vi "DB_WriteInGen.vi"(8 "error in (no error)":errorcluster, 9 "Equipo_Medicion":T2, 10 "ID_MEDICION":i32, 11 "DB in":T1) -> (0 "error out":errorcluster, 3 "closeDB":T1[](array[typedef]))   [LabVIEW 2018]
uses:
  <vilib>/addons/database/Connection.llb/Conn ObjectReference.ctl
  Controls/Equipos_Medicion_cluster.ctl
  <vilib>/addons/database/NI_Database_API.lvlib
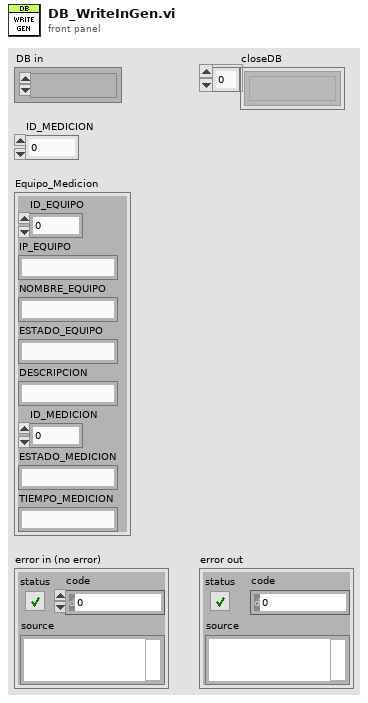
[diagram p1: front panel]
types:
  T1 = typedef "NI_Database_API.lvlib/Conn ObjectReference.ctl" = refnum<k1>
  T2 = typedef "Equipos_Medicion_cluster.ctl" = cluster{"ID_EQUIPO":i32, "IP_EQUIPO":string, "NOMBRE_EQUIPO":string, "ESTADO_EQUIPO":string, "DESCRIPCION":string, "ID_MEDICION":i32, "ESTADO_MEDICION":string, "TIEMPO_MEDICION":string}
  T3 = typedef "Cluster_Data.ctl" = cluster{"Equipo_Medicion":T2, "VIF_cluster":T4, "Power_cluster":T5, "THD_cluster":T6, "Polar_cluster":T7}
  T4 = typedef "VIF_cluster.ctl" = cluster{"VL_VL":cluster{"V1_V2":sgl, "V2_V3":sgl, "V3_V1":sgl, "Avg_VL_VL":sgl}, "IL_IL":cluster{"I1":sgl, "I2":sgl, "I3":sgl, "Avg_Amps":sgl}, "Frecuency":sgl, "Avg_Frecuency":sgl}
  T5 = typedef "Power_cluster.ctl" = cluster{"Real Power (kW)":cluster{"L1_kW":sgl, "L2_kW":sgl, "L3_kW":sgl, "Total_kW":sgl}, "Reactive Power (kVAR)":cluster{"L1_kVAR":sgl, "L2_kVAR":sgl, "L3_kVAR":sgl, "Total_kVAR":sgl}, "Aparent Power (kVA)":cluster{"L1_kVA":sgl, "L2_kVA":sgl, "L3_kVA":sgl, "Total_kVA":sgl}, "Power Factor (%)":cluster{"L1_PF":sgl, "L2_PF":sgl, "L3_PF":sgl, "Total_PF":sgl}}
  T6 = typedef "THD_cluster.ctl" = cluster{"V_THD":cluster{"Avg_V_V_THD":sgl, "V3_V1_THD":sgl, "V2_V3_THD":sgl, "V1_V2_THD":sgl}, "I_THD":cluster{"Avg_I_THD":sgl, "I4_THD":sgl, "I3_THD":sgl, "I2_THD":sgl, "I1_THD":sgl}}
  T7 = typedef "Polar_cluster.ctl" = cluster{"V_polar":cluster{"V1_ang":sgl, "V1_mag":sgl, "V2_ang":sgl, "V2_mag":sgl, "V3_ang":sgl, "V3_mag":sgl}, "I_polar":cluster{"I1_ang":sgl, "I1_mag":sgl, "I2_ang":sgl, "I2_mag":sgl, "I3_ang":sgl, "I3_mag":sgl}}
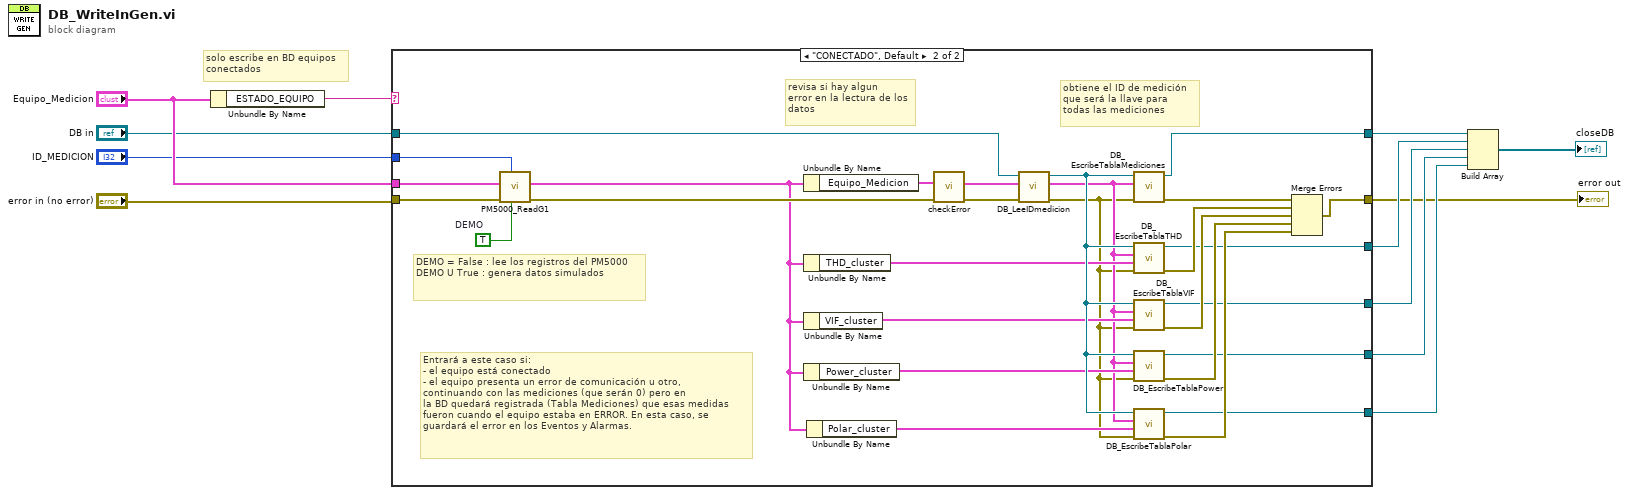
[diagram p0: block diagram]
diagram:
  # "solo escribe en BD equipos\nconectados"
  n1 = Unbundle By Name("Equipo_Medicion") -> ("ESTADO_EQUIPO"=w5:string)
  n2 = case shown="\"CONECTADO\", Default" w5 {
    tunnel: "error in (no error)" -> [w14 w42]
    tunnel: "DB in" -> [w13 w39]
    tunnel: "ID_MEDICION" -> [_ w41]
    tunnel: [w14 w38] -> w2
    tunnel: [w13 w19] -> w7
    tunnel: "Equipo_Medicion" -> [_ w40]
    tunnel: [_ w18] -> w11
    tunnel: [_ w17] -> w10
    tunnel: [_ w16] -> w9
    tunnel: [_ w15] -> w8
    frame "DESCONECTADO" {
      # "Equipo está deconectado"
    }
    frame "CONECTADO", Default {
      w36 = TRUE  # DEMO
      # "Entrará a este caso si:\n- el equipo está conectado\n- el equipo presenta un error de comunicación u otro,\ncontinuando con las mediciones (que serán 0) pero en\nla BD quedará registrada (Tabla Mediciones) que esas medidas\nfueron cuando el equipo estaba en ERROR. En esta caso, se \nguardará el error en los Eventos y Alarmas."
      # "obtiene el ID de medición\nque será la llave para \ntodas las mediciones"
      # "revisa si hay algun \nerror en la lectura de los\ndatos"
      # "DEMO = False : lee los registros del PM5000\nDEMO U True : genera datos simulados"
      n3 = call "PM5000_ReadG1.vi"("DEMO"=w36, "ID_MEDICION"=w41, "error in (no error)"=w42, "Equipo_Medicion"=w40) -> ("error out"=w37:errorcluster, "PM_out"=w35:T3)  [unwired: 6 in]
      n4 = Unbundle By Name(w35) -> ("Equipo_Medicion"=w32:T2)
      n5 = Unbundle By Name(w35) -> ("THD_cluster"=w30:T6)
      n6 = Unbundle By Name(w35) -> ("VIF_cluster"=w29:T4)
      n7 = Unbundle By Name(w35) -> ("Power_cluster"=w28:T5)
      n8 = Unbundle By Name(w35) -> ("Polar_cluster"=w26:T7)
      n9 = call "checkError.vi"("error in (no error)"=w37, "Equipo_Medicion in"=w32) -> ("error out"=w34:errorcluster, "Equipo_Medicion out"=w31:T2)  [unwired: 8 in]
      n10 = call "DB_LeeIDmedicion.vi"("error in (no error)"=w34, "Equipo_Medicion in"=w31, "db in"=w39) -> ("error out"=w25:errorcluster, "Equipo_Medicion out"=w27:T2, "db out"=w33:T1)  [unwired: 6 in]
      n11 = call "DB_EscribeTablaMediciones.vi"("error in (no error)"=w25, "Equipo_Medicion in"=w27, "db in"=w33) -> ("error out"=w24:errorcluster, "db out"=w19:T1)  [unwired: 7 in]
      n12 = call "DB_EscribeTablaTHD.vi"("error in (no error)"=w25, "THD_cluster"=w30, "Equipo_Medicion"=w27, "db in"=w33) -> ("error out"=w23:errorcluster, "db out"=w15:T1)  [unwired: 6 in]
      n13 = call "DB_EscribeTablaVIF.vi"("error in (no error)"=w25, "VIF_cluster"=w29, "Equipo_Medicion"=w27, "db in"=w33) -> ("error out"=w22:errorcluster, "db out"=w16:T1)  [unwired: 6 in]
      n14 = call "DB_EscribeTablaPower.vi"("error in (no error)"=w25, "Power_cluster"=w28, "Equipo_Medicion"=w27, "db in"=w33) -> ("error out"=w21:errorcluster, "db out"=w17:T1)  [unwired: 6 in]
      n15 = call "DB_EscribeTablaPolar.vi"("error in (no error)"=w25, "Polar_cluster"=w26, "Equipo_Medicion"=w27, "db in"=w33) -> ("error out"=w20:errorcluster, "db out"=w18:T1)  [unwired: 6 in]
      n16 = Merge Errors(w24, w23, w22, w21, w20) -> (w38:errorcluster)
    }
  }
  "error out" <- w2
  n17 = Build Array(w7, w8, w9, w10, w11) -> (→"closeDB":T1[])
